vi "QSM_MAIN.vi"(8 "Error In":errorcluster, 11 "QSM_ShiftRegister in":T1) -> (0 "Error Out":errorcluster, 3 "QSM_ShiftRegister out":T1)   [LabVIEW 2014, in "GUIUpdateQSM.lvlib"]
doc: "The Display Update (DISP.UPDT) Queued State Machine (QSM) handles configuration Pop-Up windows and control updates on the main application interface."
uses:
  GUIUpdateQSM.lvlib
  Controls/QSM_ShiftRegister.ctl
  QueueMaintenance/TypeDef/QSMRef_ALL.ctl
  Controls/QSM_Reference.ctl
  Controls/QSM_DataType.ctl
  Controls/QSM_RunStates.ctl
  Queue_TEST/Controls/QSM_Reference.ctl
  Queue_TEST/Controls/QSM_DataType.ctl
  Queue_TEST/Controls/QSM_RunStates.ctl
  Controls/TypeDef_FrontPanelReferences.ctl
  QueueMaintenance/QueueMaintenance.lvlib
  Queue_TEST/TestQSM.lvlib
panel:
  # "MAIN QSM - Update GUI"
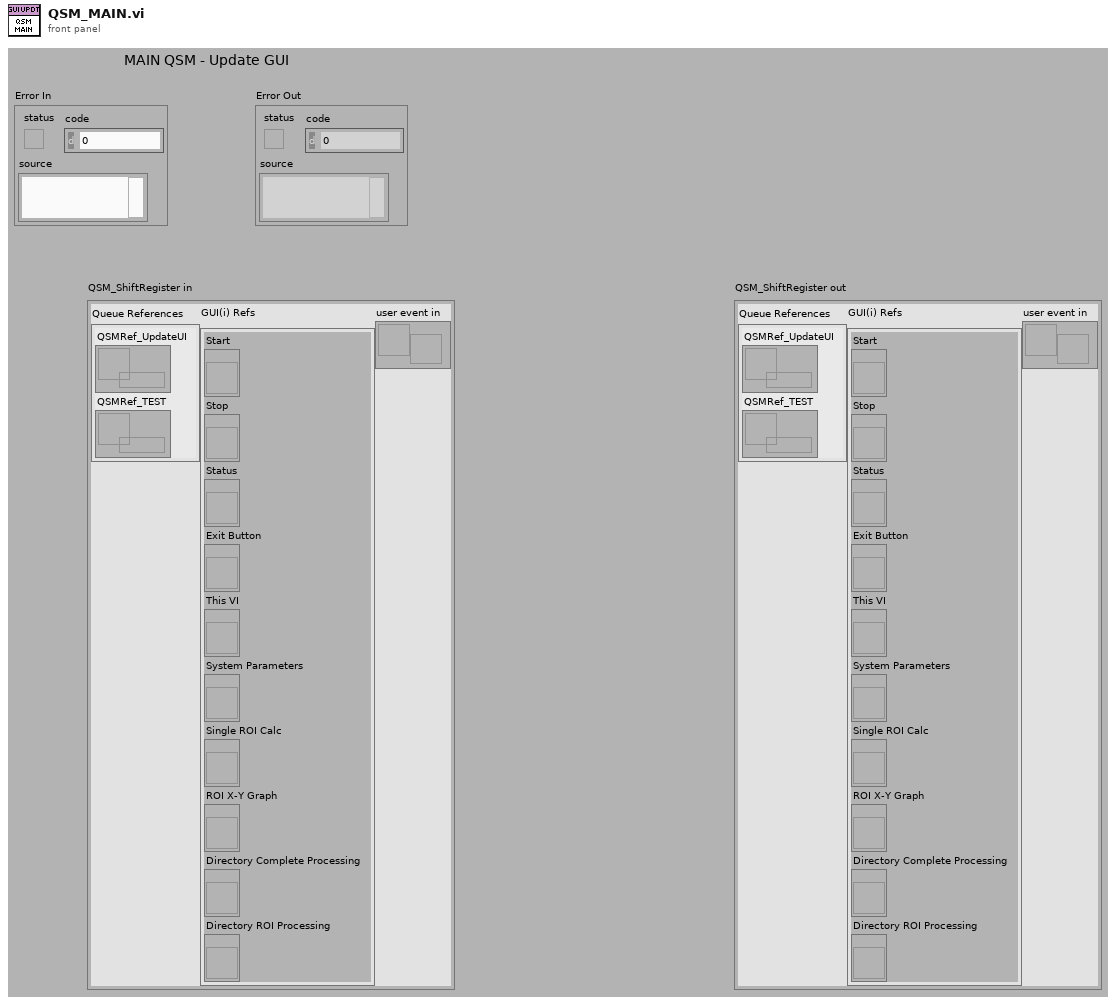
[diagram p1: front panel]
types:
  T1 = typedef "GUIUpdateQSM.lvlib/QSM_ShiftRegister.ctl" = cluster{"Queue References":T2, "GUI(i) Refs":T5, "user event in":refnum<user-event>}
  T2 = typedef "QueueMaintenance.lvlib/QSMRef_ALL.ctl" = cluster{"QSMRef_UpdateUI":T3, "QSMRef_TEST":T4}
  T3 = typedef "GUIUpdateQSM.lvlib/QSM_Reference.ctl" = refnum<queue>
  T4 = typedef "TestQSM.lvlib/QSM_Reference.ctl" = refnum<queue>
  T5 = typedef "GUIUpdateQSM.lvlib/TypeDef_FrontPanelReferences.ctl" = cluster{"Start":refnum<vi>, "Stop":refnum<vi>, "Status":refnum<vi>, "Exit Button":refnum<vi>, "This VI":refnum<vi>, "System Parameters":refnum<vi>, "Single ROI Calc":refnum<vi>, "ROI X-Y Graph":refnum<vi>, "Directory Complete Processing":refnum<vi>, "Directory ROI Processing":refnum<vi>}
  T6 = typedef "GUIUpdateQSM.lvlib/QSM_RunStates.ctl" = enum16{"NULL", "Sect01_Initialize-00_GROUP.ENQUEUE", "Sect01_Initialize-01_SetMainToDefault", "Sect01_Initialize-02_Clear Status Strings", "Sect02_UpdateUI-00_Enable Stop_ Disable Start", "Sect02_UpdateUI-01_Enable Start_Disable Stop", "Sect02_UpdateUI-02_Update Status String", "Sect02_UpdateUI-03_Clear XY-Graph", "Sect03-Open ROI  GUI", "Sect03-Close ROI GUI", "Sect99_EXIT-00_Group.Enqueue", "Sect99_EXIT-01_CloseReferences", "Sect99_EXIT-02_StopQSM"}
  T7 = typedef "GUIUpdateQSM.lvlib/QSM_DataType.ctl" = cluster{"QSM_RunStates":T6, "DATA.VARIANT":variant}
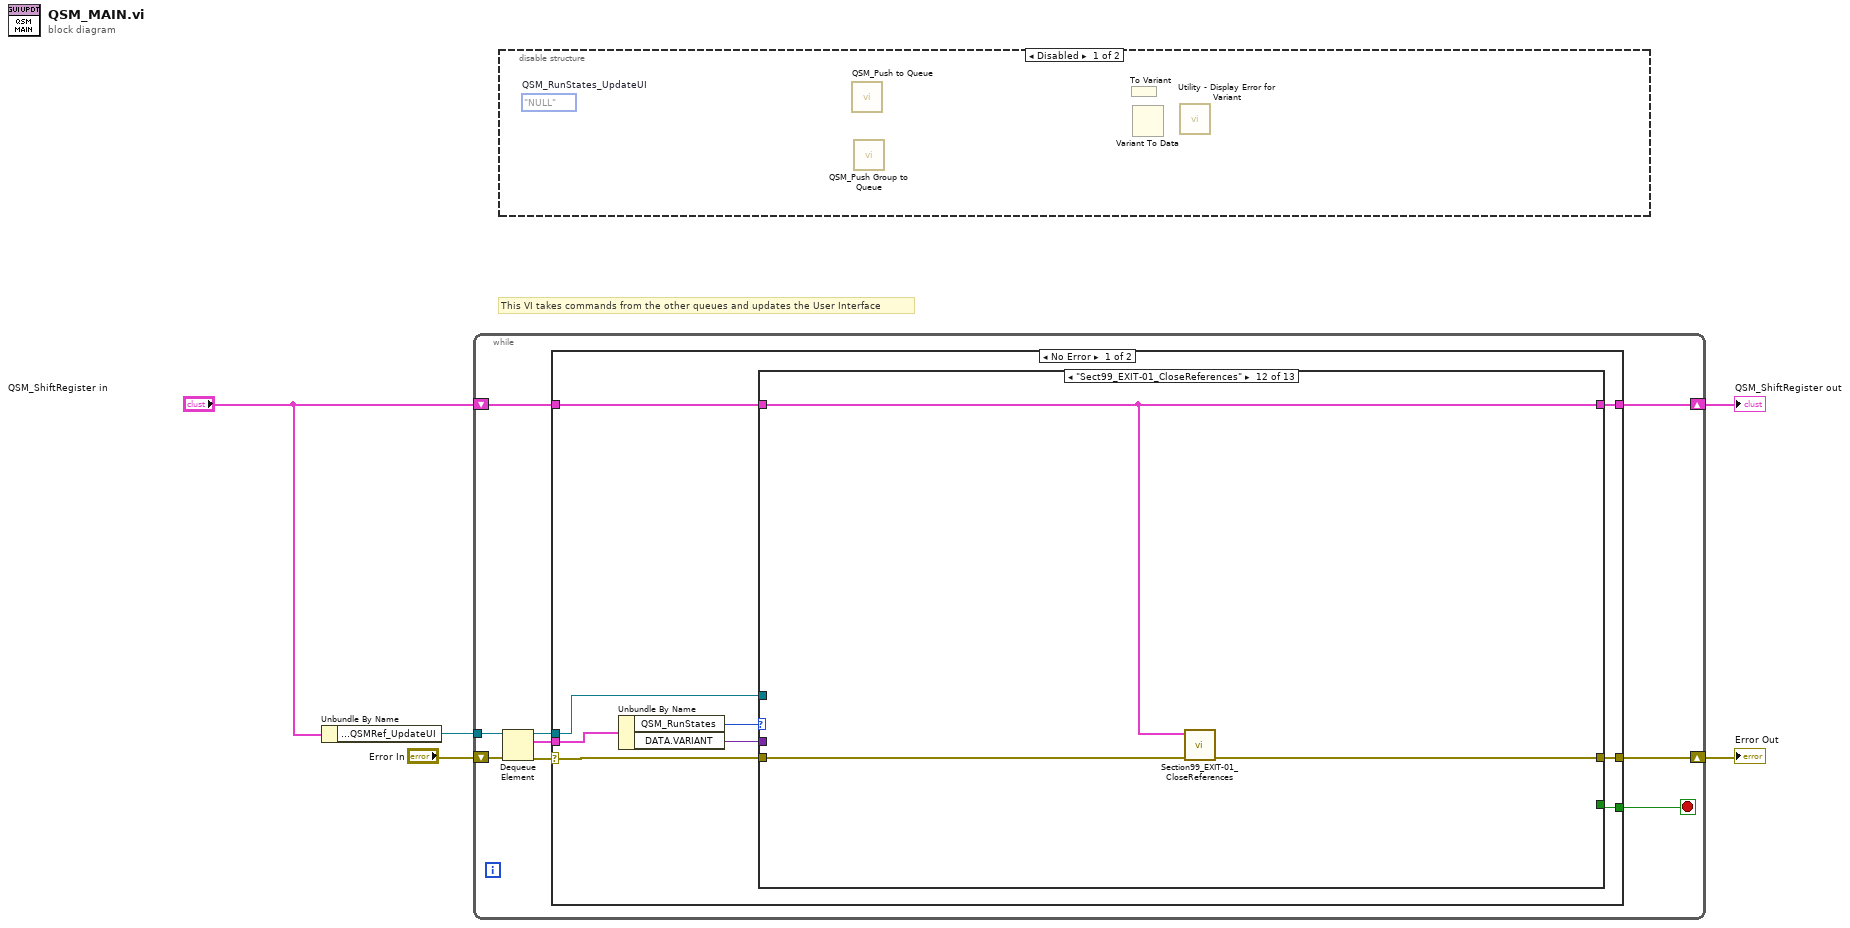
[diagram p0: block diagram]
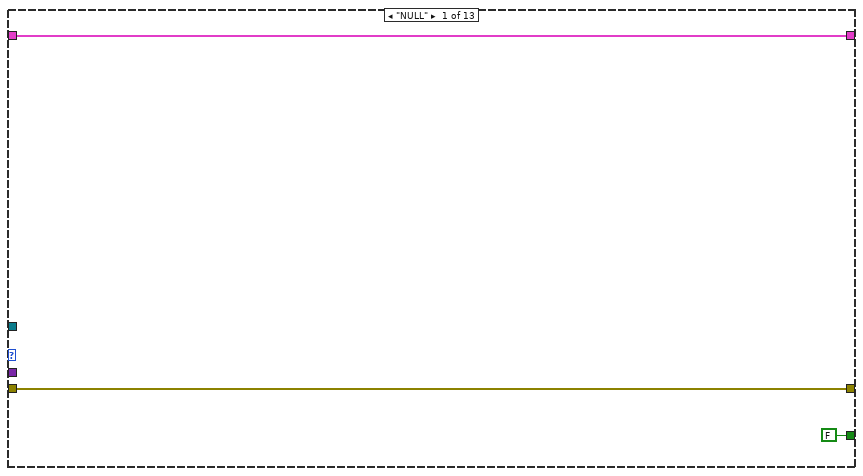
[diagram p3: hidden frame]
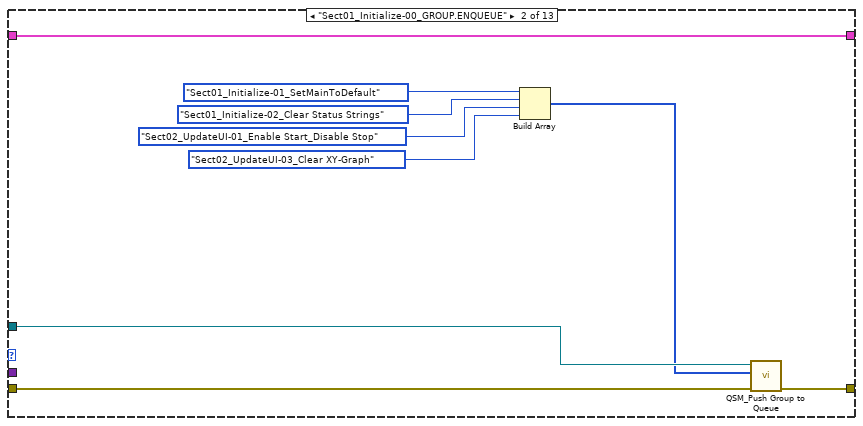
[diagram p4: hidden frame]
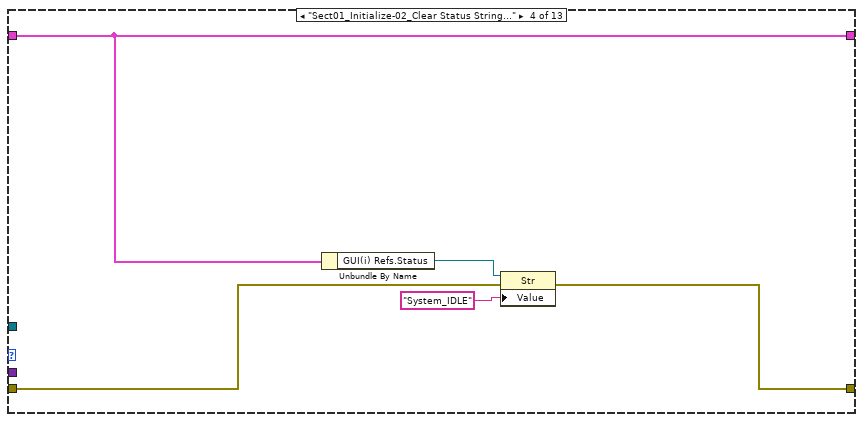
[diagram p6: hidden frame]
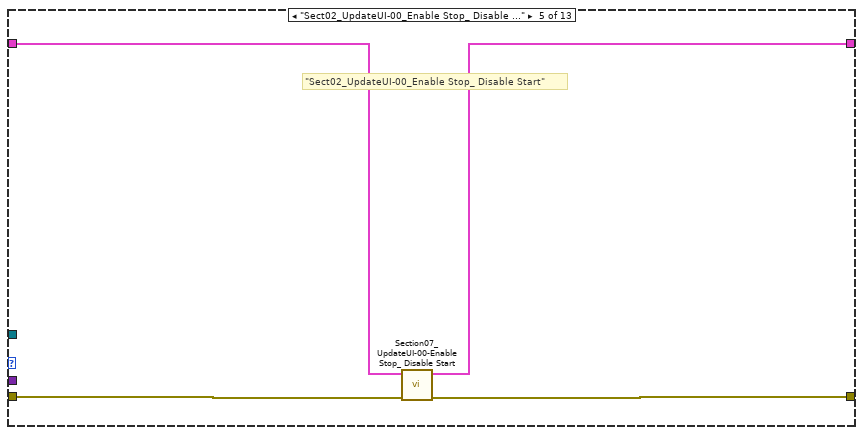
[diagram p7: hidden frame]
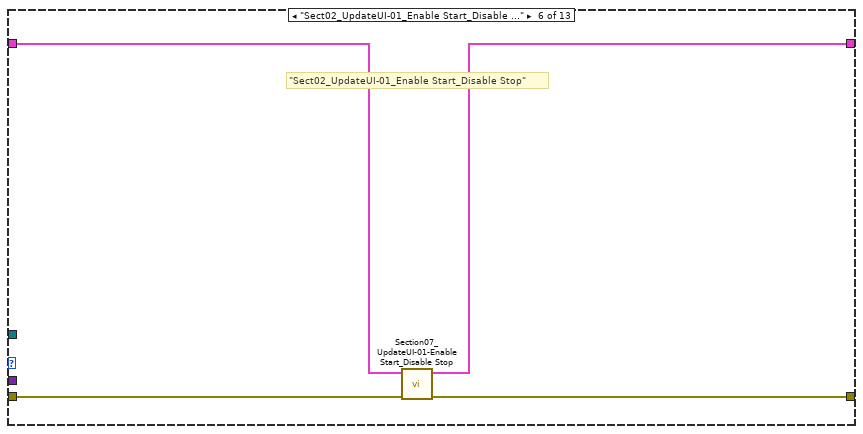
[diagram p8: hidden frame]
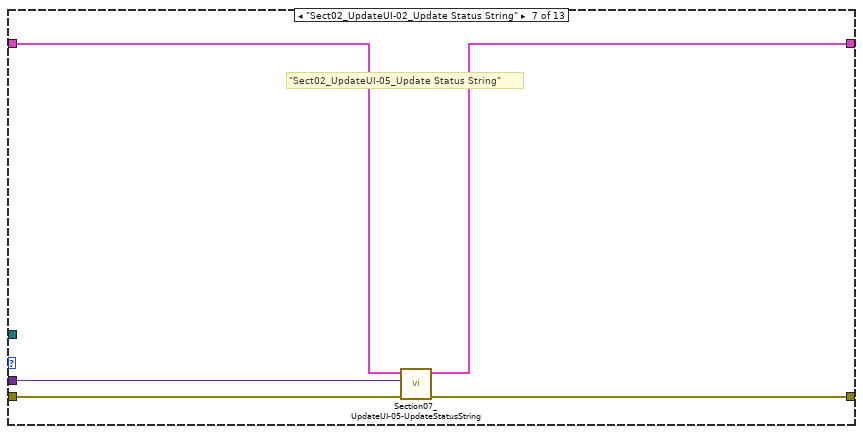
[diagram p9: hidden frame]
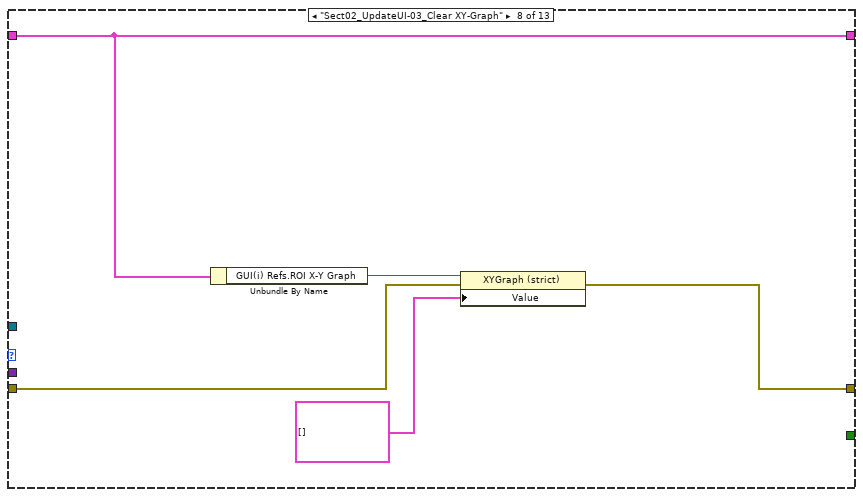
[diagram p10: hidden frame]
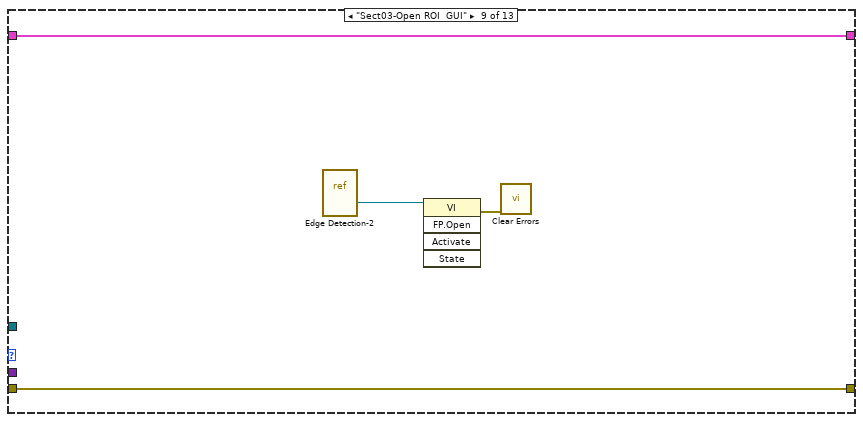
[diagram p11: hidden frame]
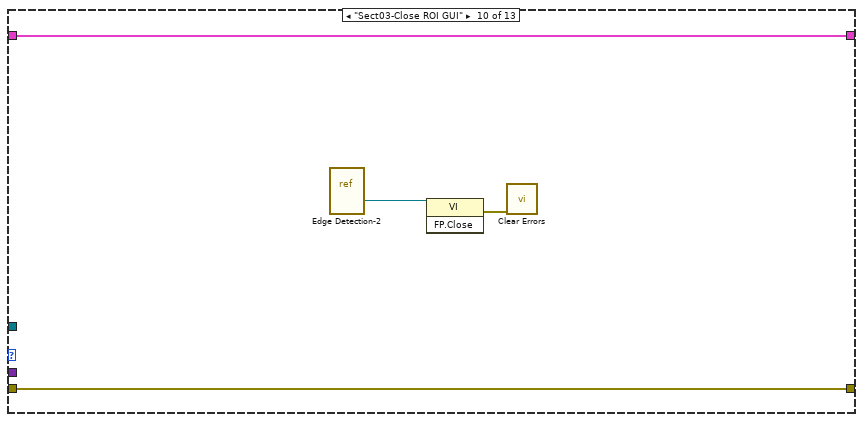
[diagram p12: hidden frame]
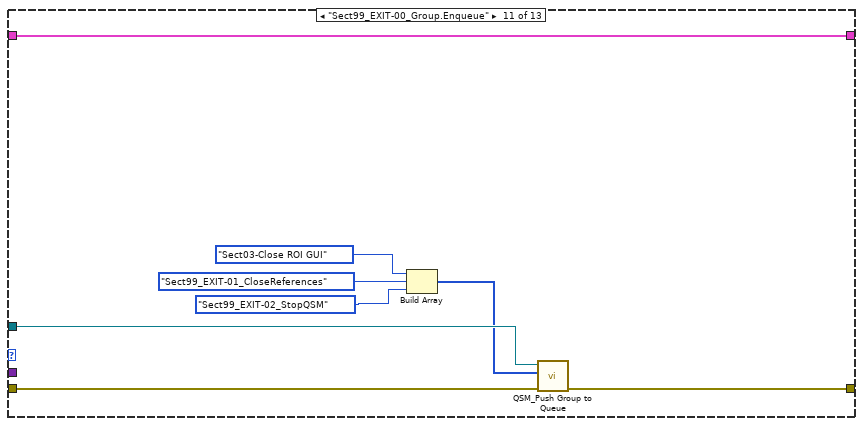
[diagram p13: hidden frame]
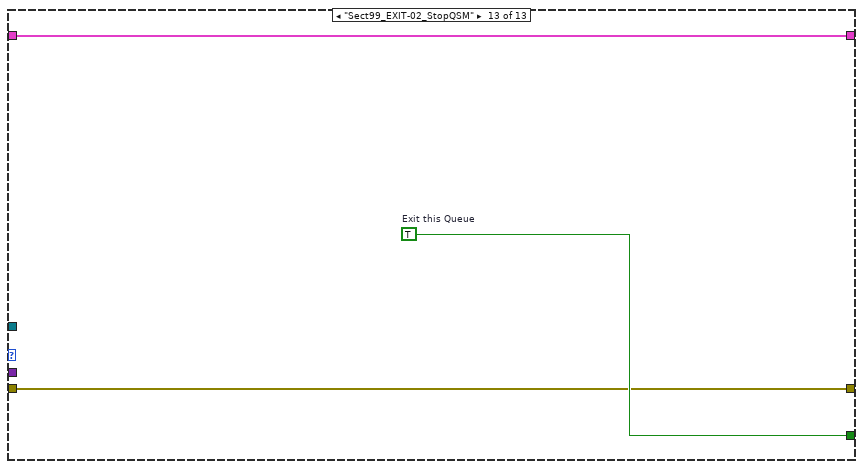
[diagram p14: hidden frame]
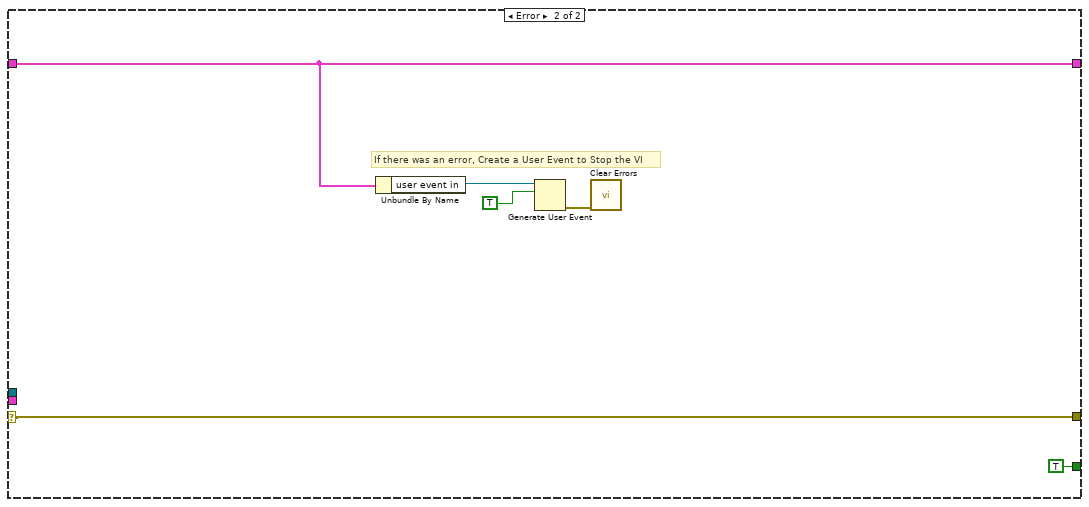
[diagram p15: hidden frame]
diagram:
  # "This VI takes commands from the other queues and updates the User Interface"
  n1 = Unbundle By Name("QSM_ShiftRegister in") -> ("Queue References.QSMRef_UpdateUI"=w3:T3)
  n2 = while {
    tunnel: w3 -> [w13]
    shift-right: [w11] -> w2
    shift-left: "QSM_ShiftRegister in" -> [w10]
    shift-right: [w6] -> w4
    shift-left: "Error In" -> [w14]
    stop <- w9 stop-if-true
    n3 = Dequeue Element(queue=w13, error in (no error)=w14) -> (queue out=w8:T3, element=w12:T7, error out=w7:errorcluster)  [unwired: 1 in, 1 out]
    n4 = case shown="No Error" w7 {
      selector: w7 -> [w15 w88]
      tunnel: w12 -> [w23 _]
      tunnel: [w20 w88] -> w6
      tunnel: [w19 w83] -> w11
      tunnel: w10 -> [w18 w83]
      tunnel: [w17 TRUE ("Exit this Queue")] -> w9
      tunnel: w8 -> [w16 _]
      frame No Error {
        n5 = Unbundle By Name(w23) -> ("QSM_RunStates"=w22:T6, "DATA.VARIANT"=w21:variant)
        n6 = case shown="\"Sect99_EXIT-01_CloseReferences\"" w22 {
          tunnel: w15 -> [w26 w33 w36 w38 w44 w48 w52 w57 w64 w68 w75 w78 w80]
          tunnel: w21 -> [_ _ _ _ _ _ w51 _ _ _ _ _ _]
          tunnel: [w26 w34 w36 w41 w43 w47 w53 w59 w64 w68 w74 w79 w80] -> w20
          tunnel: w18 -> [w25 w35 w37 w39 w46 w50 w55 w58 w63 w67 w76 w77 w82]
          tunnel: [w25 w35 w37 w39 w45 w49 w54 w58 w63 w67 w76 w77 w82] -> w19
          tunnel: [FALSE _ _ _ _ _ _ _ _ _ _ _ w81] -> w17
          tunnel: w16 -> [_ w32 _ _ _ _ _ _ _ _ w73 _ _]
          frame "NULL" {
          }
          frame "Sect01_Initialize-00_GROUP.ENQUEUE" {
            n7 = Build Array(QSM_RunStates."Sect01_Initialize-01_SetMainToDefault" ("QSM_RunStates_UpdateUI"), QSM_RunStates."Sect01_Initialize-02_Clear Status Strings" ("QSM_RunStates_UpdateUI"), QSM_RunStates."Sect02_UpdateUI-01_Enable Start_Disable Stop" ("QSM_RunStates_UpdateUI"), QSM_RunStates."Sect02_UpdateUI-03_Clear XY-Graph" ("QSM_RunStates_UpdateUI")) -> (w29:T6[])
            n8 = call "QSM_Push Group to Queue.vi"("error in (no error)"=w33, "Group Cmds to Push"=w29, "QSMRef in"=w32) -> ("error out"=w34:errorcluster)  [unwired: 7 in, 1 out]
          }
          frame "Sect01_Initialize-01_SetMainToDefault" {
            # "Empty Case left for future expansion"
          }
          frame "Sect01_Initialize-02_Clear Status Strings" {
            n9 = Unbundle By Name(w39) -> ("GUI(i) Refs.Status"=w42:refnum<vi>)
            n10 = property class="Str"(reference=w42, error in=w38, "Value"="System_IDLE") -> (error out=w41:errorcluster)  [unwired: 1 out]
          }
          frame "Sect02_UpdateUI-00_Enable Stop_ Disable Start" {
            # "\"Sect02_UpdateUI-00_Enable Stop_ Disable Start\""
            n11 = call "Section07_UpdateUI-00-Enable Stop_ Disable Start.vi"("error in (no error)"=w44, "ShiftRegister in"=w46) -> ("error out"=w43:errorcluster, "ShiftRegister out"=w45:T1)  [unwired: 8 in]
          }
          frame "Sect02_UpdateUI-01_Enable Start_Disable Stop" {
            # "\"Sect02_UpdateUI-01_Enable Start_Disable Stop\""
            n12 = call "Section07_UpdateUI-01-Enable Start_Disable Stop.vi"("error in (no error)"=w48, "QSM_ShiftRegister  in"=w50) -> ("error out"=w47:errorcluster, "QSM_ShiftRegister out"=w49:T1)  [unwired: 8 in]
          }
          frame "Sect02_UpdateUI-02_Update Status String" {
            # "\"Sect02_UpdateUI-05_Update Status String\""
            n13 = call "Section07_UpdateUI-05-UpdateStatusString.vi"("error in (no error)"=w52, "Variant Data"=w51, "QSM_ShiftRegister_UpdateUI_In in"=w55) -> ("error out"=w53:errorcluster, "QSM_ShiftRegister_UpdateUI_In out"=w54:T1)  [unwired: 7 in]
          }
          frame "Sect02_UpdateUI-03_Clear XY-Graph" {
            n14 = Unbundle By Name(w58) -> ("GUI(i) Refs.ROI X-Y Graph"=w60:refnum<vi>)
            n15 = property class="XYGraph (strict)"(reference=w60, error in=w57, "Value"=cluster{"X":dbl[], "Y":dbl[]}[] []) -> (error out=w59:errorcluster)  [unwired: 1 out]
          }
          frame "Sect03-Open ROI  GUI" {
            n16 = vi-ref "Edge Detection-2.vi"() -> (w62:refnum<vi>)
            n17 = invoke class="VI" method="FP.Open"(reference=w62) -> (error out=w61:errorcluster)  [unwired: 4 in, 4 out]
            n18 = call <vilib>:"Clear Errors.vi"("error in (no error)"=w61) -> ()  [unwired: 5 in, 2 out]
          }
          frame "Sect03-Close ROI GUI" {
            n19 = vi-ref "Edge Detection-2.vi"() -> (w66:refnum<vi>)
            n20 = invoke class="VI" method="FP.Close"(reference=w66) -> (error out=w65:errorcluster)  [unwired: 2 in, 2 out]
            n21 = call <vilib>:"Clear Errors.vi"("error in (no error)"=w65) -> ()  [unwired: 5 in, 2 out]
          }
          frame "Sect99_EXIT-00_Group.Enqueue" {
            n22 = Build Array(QSM_RunStates."Sect03-Close ROI GUI" ("QSM_RunStates_UpdateUI"), QSM_RunStates."Sect99_EXIT-01_CloseReferences" ("QSM_RunStates_UpdateUI"), QSM_RunStates."Sect99_EXIT-02_StopQSM" ("QSM_RunStates_UpdateUI")) -> (w70:T6[])
            n23 = call "QSM_Push Group to Queue.vi"("error in (no error)"=w75, "Group Cmds to Push"=w70, "QSMRef in"=w73) -> ("error out"=w74:errorcluster)  [unwired: 7 in, 1 out]
          }
          frame "Sect99_EXIT-01_CloseReferences" {
            n24 = call "Section99_EXIT-01_CloseReferences.vi"("error in (no error)"=w78, "ShiftRegister in"=w77) -> ("error out"=w79:errorcluster)  [unwired: 9 in]
          }
          frame "Sect99_EXIT-02_StopQSM" {
            w81 = TRUE  # Exit this Queue
          }
        }
      }
      frame Error {
        # "If there was an error, Create a User Event to Stop the VI"
        n25 = Unbundle By Name(w83) -> ("user event in"=w86:refnum<user-event>)
        n26 = Generate User Event(user event=w86, event data cluster=TRUE ("event data")) -> (error out=w84:errorcluster)  [unwired: 2 in, 1 out]
        n27 = call <vilib>:"Clear Errors.vi"("error in (no error)"=w84) -> ()  [unwired: 5 in, 2 out]
      }
    }
  }
  "Error Out" <- w4
  "QSM_ShiftRegister out" <- w2
  n28 = disable-structure shown="Disabled" {
    frame Disabled {
      (unwired) QSM_RunStates."NULL"  # QSM_RunStates_UpdateUI
      n29 = call "QSM_Push to Queue.vi"() -> ()  [unwired: 10 in, 2 out]
      n30 = call "QSM_Push Group to Queue.vi"() -> ()  [unwired: 10 in, 2 out]
      n31 = To Variant() -> ()  [unwired: 1 in, 1 out]
      n32 = Variant To Data() -> ()  [unwired: 3 in, 2 out]
      n33 = call "Utility - Display Error for Variant.vi"() -> ()  [unwired: 11 in, 1 out]
    }
    frame Enabled {
    }
  }
